vi "Intake Forever_wrapper.vi"(10 "Setpoint":dbl) -> ()   [LabVIEW 2019]
uses:
  <vilib>/Rock Robotics/WPI/Framework/Completion Status.ctl
  <vilib>/Rock Robotics/WPI/Framework/Completion Notifier.ctl
  <vilib>/Rock Robotics/WPI/Framework/Command Status Info.ctl
panel:
  out "Command Info Out":T1
  in  "Command Info In":T1
  in  "Description":string
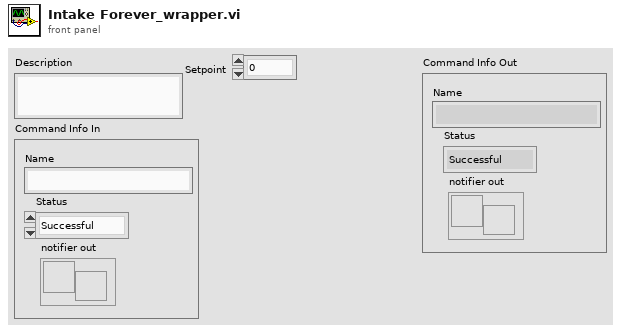
[diagram p1: front panel]
types:
  T1 = typedef "Command Status Info.ctl" = cluster{"Name":string, "Status":T2, "notifier out":T3}
  T2 = typedef "Completion Status.ctl" = enum16{"Successful", "Aborted", "Incomplete"}
  T3 = typedef "Completion Notifier.ctl" = refnum<notifier>
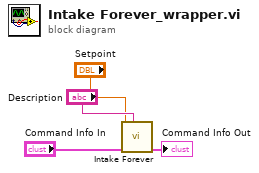
[diagram p0: block diagram]
diagram:
  n1 = call "Intake Forever.vi"("Description"="Description", "Command Info In"="Command Info In", "Setpoint"="Setpoint") -> ("Command Info Out"=→"Command Info Out":T1)  [unwired: 8 in]
